vi "Timing_AnalogOut.vi"() -> ()   [LabVIEW 2016]
uses:
  <vilib>/Platform/TimedLoop/XDataNode/timing_clust.ctl
  <vilib>/Platform/TimedLoop/XDataNode/nitl_modes.ctl
  <vilib>/Platform/TimedLoop/XDataNode/wakeup.ctl
  <vilib>/rvi/Emulation/niFpgaGetClockAttributes.vi
  <vilib>/rvi/Emulation/niFpgaSctlEmulationGetInTimedLoop.vi
  <vilib>/rvi/Emulation/niFpgaEmulationReportErrorSimple.vi
  <vilib>/rvi/Emulation/niFpgaCriticalErrorInLSC.vi
  <vilib>/rvi/eio/common/nirviEmuTemplateMethod_errors.vi
  <vilib>/Platform/TimedLoop/XDataNode/XDataNode.xnode
  <vilib>/eio/EIONode/EIONode.xnode
  <vilib>/Platform/TimedLoop/XDataNode/XDNodeRunTimeDep.lvlib
panel:
  in  "Samples Y":i16=3
  in  "Flip axis?":bool
  in  "Offset Y":i16
  in  "Scale Y":i16
  in  "Samples X":i16=3
  in  "Offset X":i16
  in  "Scale X":i16
  out "Laser clock (ticks)":u32=64
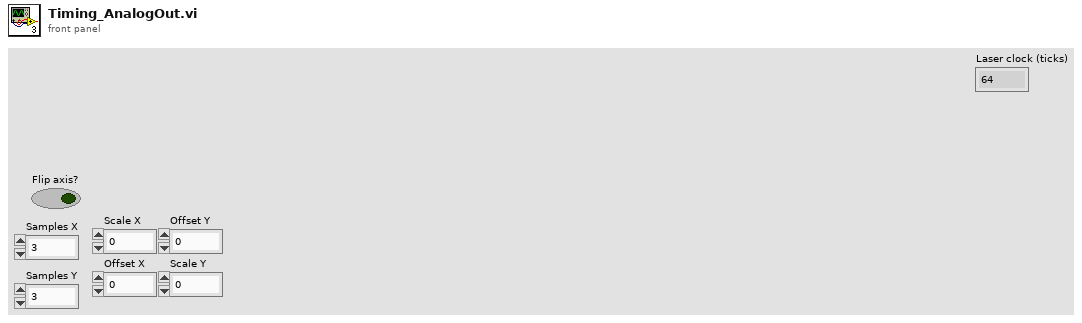
[diagram p1: front panel]
types:
  T1 = typedef "XDNodeRunTimeDep.lvlib/timing_clust.ctl" = cluster{"Expected End [f-1]":u64, "Actual End [f-1]":u64, "Finished Late? [f-1]":bool, "Expected End [i-1]":u64, "Actual End [i-1]":u64, "Finished Late? [i-1]":bool, "Expected Start [i]":u64, "Actual Start [i]":u64, "Expected Start [f]":u64, "Actual Start [f]":u64, "Source Name":string, "Structure Name":string, "Period":i64, "Deadline":i64, "Offset":i64, "Start":i64, "Priority":i32, "Timeout":i32, "Mode":T2, "Wakeup Reason":T3, "Error":errorcluster, "Source Type":string, "Secondary Source Type":string, "Global End Time":u64, "Global Start Time":u64, "Frame Duration":u64, "Iteration Duration":u64, "Assigned CPU":i32, "I/O Scan Engine Mode":u32}
  T2 = typedef "XDNodeRunTimeDep.lvlib/nitl_modes.ctl" = enum32{"No Change", "Process missed periods, maintain original phase", "Discard missed periods, maintain original phase", "Process missed periods, ignore original phase", "Discard missed periods, ignore original phase"}
  T3 = typedef "XDNodeRunTimeDep.lvlib/wakeup.ctl" = enum32{"Normal", "Aborted", "Asynchronous wakeup", "Timing source error", "Timed loop error", "Timeout"}
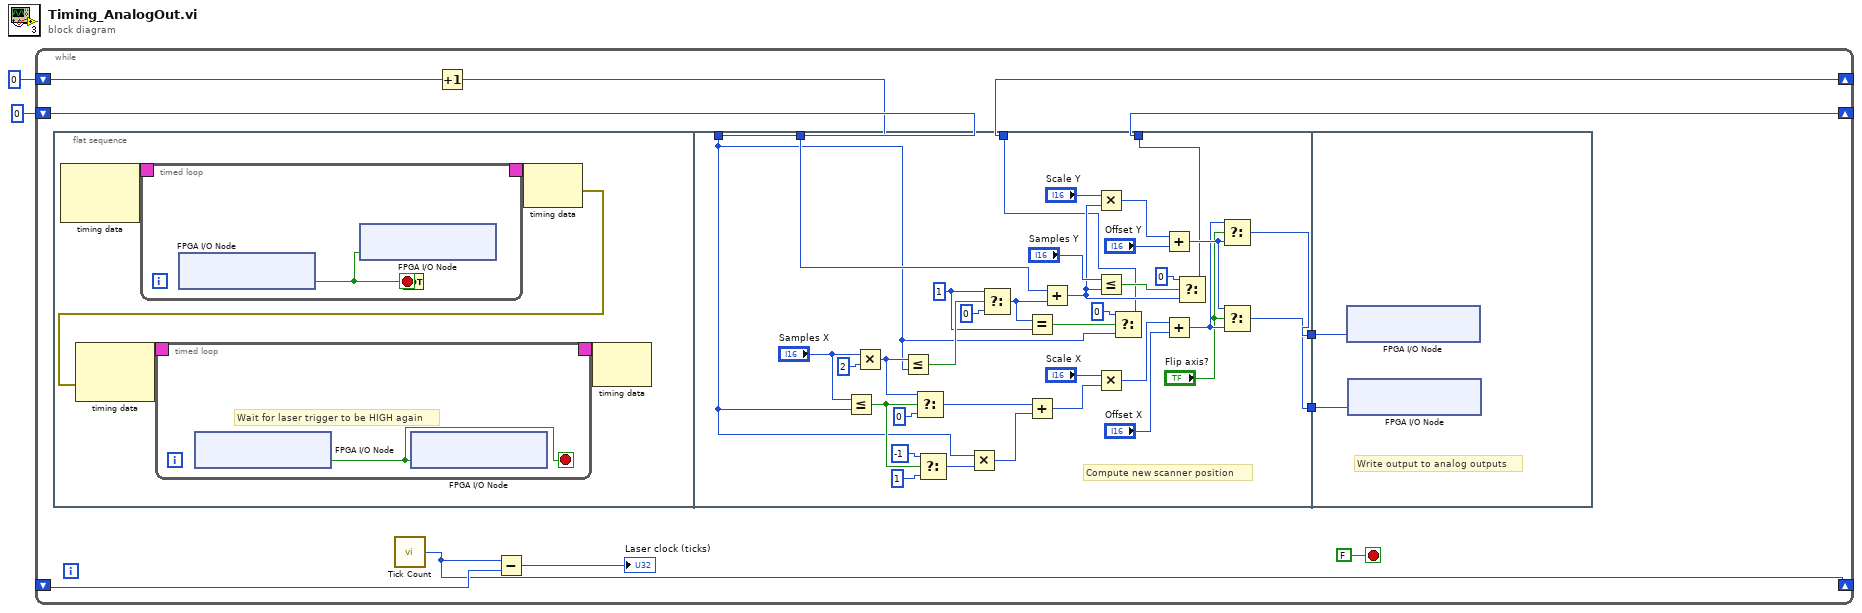
[diagram p0: block diagram]
diagram:
  n1 = while {
    shift-right: [w11] -> _
    shift-left: _ -> [w12]
    shift-right: [w4] -> _
    shift-left: i16 0 -> [w5]
    shift-right: [w7] -> _
    shift-left: i16 0 -> [w6]
    stop <- FALSE ("stop") stop-if-true
    n2 = flat-sequence {
      tunnel: [w60] -> w9
      tunnel: [w59] -> w8
      tunnel: [w55] -> w7
      tunnel: w3 -> [w33]
      tunnel: w6 -> [w50]
      tunnel: [w44] -> w4
      tunnel: w9 -> [w70]
      tunnel: w8 -> [w69]
      frame #0 {
        n3 = node-c288() -> (w18:T1)  [unwired: 2 in]
        n4 = timed-loop {
          timing: w18 -> [_]
          timing-out: [_] -> w17
          stop <- w26 stop-if-true
          n5 = xnode "FPGA I/O Node"() -> ("Connector0/DIO4"=w27:bool)  [unwired: 1 in, 1 out]
          n6 = xnode "FPGA I/O Node"("Connector0/DIO0"=w27) -> ()  [unwired: 1 in, 1 out]
          n7 = Not(x=w27) -> (.not. x?=w26:bool)
        }
        n8 = node-c288(w17) -> (w14:errorcluster)
        n9 = node-c288(w14) -> (w16:T1)  [unwired: 1 in]
        n10 = timed-loop {
          timing: w16 -> [_]
          timing-out: [_] -> w15
          stop <- w19 stop-if-true
          # "Wait for laser trigger to be HIGH again"
          n11 = xnode "FPGA I/O Node"() -> ("Connector0/DIO4"=w19:bool)  [unwired: 1 in, 1 out]
          n12 = xnode "FPGA I/O Node"("Connector0/DIO0"=w19) -> ()  [unwired: 1 in, 1 out]
        }
        n13 = node-c288(w15) -> ()  [unwired: 1 out]
      }
      frame #1 {
        w47 = i16 1 ("t")
        # "Compute new scanner position"
        n14 = Less Or Equal?(x="Samples X", y=w33) -> (x <= y?=w40:bool)
        n15 = Multiply(x="Samples X", y=i16 2) -> (x*y=w38:i16)
        n16 = Less Or Equal?(x=w38, y=w33) -> (x <= y?=w52:bool)
        n17 = Select(t=w38, s=w40, f=i16 0) -> (s? t:f=w37:i16)
        n18 = Select(t=i16 -1, s=w40, f=i16 1) -> (s? t:f=w34:i16)
        n19 = Multiply(x=w33, y=w34) -> (x*y=w36:i16)
        n20 = Select(t=w47, s=w52, f=i16 0) -> (s? t:f=w48:i16)
        n21 = Equal?(x=w48, y=w47) -> (x = y?=w46:bool)
        n22 = Add(x=w37, y=w36) -> (x+y=w35:i16)
        n23 = Add(x=w50, y=w48) -> (x+y=w49:i16)
        n24 = Multiply(x="Scale Y", y=w49) -> (x*y=w64:i16)
        n25 = Less Or Equal?(x="Samples Y", y=w49) -> (x <= y?=w57:bool)
        n26 = Multiply(x="Scale X", y=w35) -> (x*y=w67:i16)
        n27 = Select(t=i16 0 ("f"), s=w46, f=w33) -> (s? t:f=w44:i16)
        n28 = Add(x=w64, y="Offset Y") -> (x+y=w63:i16)
        n29 = Add(x=w67, y="Offset X") -> (x+y=w62:i16)
        n30 = Select(t=i16 0, s=w57, f=w49) -> (s? t:f=w55:i16)
        n31 = Select(t=w62, s="Flip axis?", f=w63) -> (s? t:f=w60:i16)
        n32 = Select(t=w63, s="Flip axis?", f=w62) -> (s? t:f=w59:i16)
      }
      frame #2 {
        # "Write output to analog outputs"
        n33 = xnode "FPGA I/O Node"("Connector0/AO0"=w70) -> ()  [unwired: 1 in, 1 out]
        n34 = xnode "FPGA I/O Node"("Connector0/AO1"=w69) -> ()  [unwired: 1 in, 1 out]
      }
    }
    n35 = call "Tick Count"() -> ("Tick Count(Ticks)"=w11:u32)
    n36 = Increment(x=w5) -> (x+1=w3:i16)
    n37 = Subtract(x=w11, y=w12) -> (x-y=→"Laser clock (ticks)":u32)
  }
